vi "List Categories.vi"(8 "error in (no error)":errorcluster, 11 "JKI SM in":refnum<class "JKI SM.lvclass">) -> (0 "error out":errorcluster, 1 "Frame Indices":i32[](array[numeric]), 2 "All State Categories":string[](array[string]), 3 "JKI SM out":refnum<class "JKI SM.lvclass">)   [LabVIEW 2020, in "JKI State Machine API.lvlib" / "JKI SM.lvclass"]
uses:
  JKI SM.lvclass
  JKI SM.lvclass/JKI SM.ctl
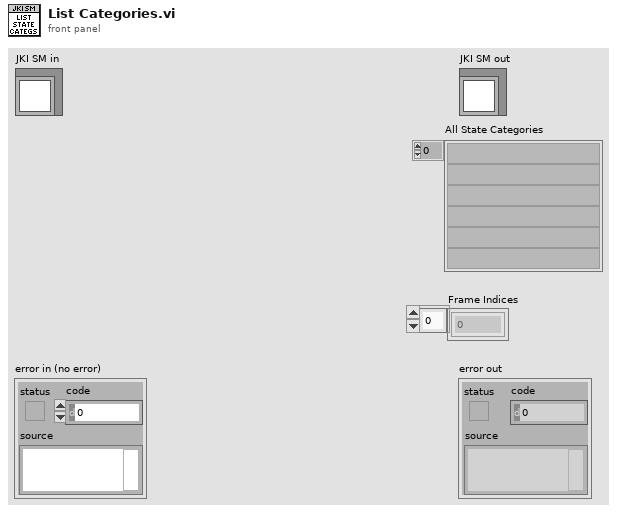
[diagram p1: front panel]
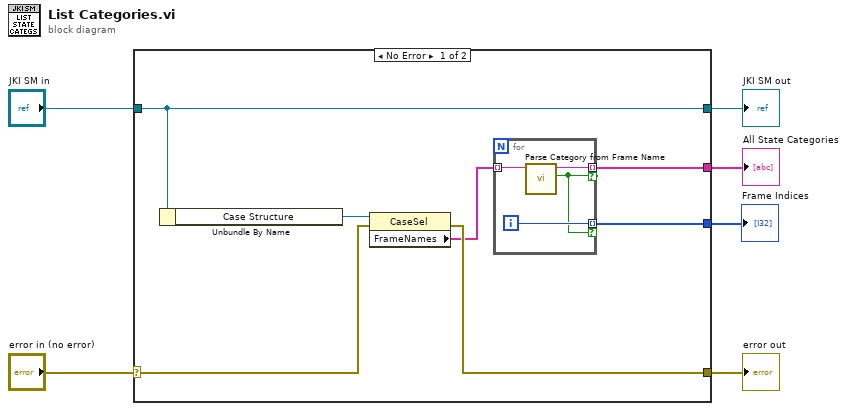
[diagram p0: block diagram]
diagram:
  n1 = case shown="No Error" "error in (no error)" {
    selector: "error in (no error)" -> [w11 w19]
    tunnel: [w10 w19] -> w5
    tunnel: [w13 w18] -> w3
    tunnel: "JKI SM in" -> [w13 w18]
    tunnel: [w8 _] -> w2
    tunnel: [w7 _] -> w1
    frame No Error {
      n2 = Unbundle By Name(w13) -> ("Case Structure"=w12:refnum<vi>)
      n3 = property class="CaseSel"(reference=w12, error in=w11) -> (error out=w10:errorcluster, "FrameNames"=w9:string[])  [unwired: 1 out]
      n4 = for {
        tunnel: w9 -> [w17] mode=indexing
        tunnel: [w16] -> w8 mode=indexing if=w14
        tunnel: [w15] -> w7 mode=indexing if=w14
        i -> [w15]
        n5 = call "Parse Category from Frame Name.vi"("Frame Name"=w17) -> ("is a Category?"=w14:bool, "Category Name"=w16:string)  [unwired: 9 in]
      }
    }
    frame Error {
    }
  }
  "error out" <- w5
  "JKI SM out" <- w3
  "All State Categories" <- w2
  "Frame Indices" <- w1
